vi "OuputMixer5782_500Mhz_2channel.vi"(6 "reset":bool, 8 "valid in":bool, 9 "Sine in":fxp<+/-,16,0>[](array[numeric])=[0.0, 0.0, 0.0, 0.0], 10 "Cosine in":fxp<+/-,16,0>[](array[numeric])=[0.0, 0.0, 0.0, 0.0], 11 "Data in":fxp<+/-,16,14>[](array[numeric])=[0.0, 0.0]) -> (0 "valid out":bool, 3 "appended array":i16[](array[numeric]))   [LabVIEW 2013]
doc: "Outputs input from channel 0 as I*cos(t)-Q*sin(t) on analog output 0"
uses:
  <vilib>/eio/EIONode/EIONode.xnode
  <vilib>/rvi/eio/common/nirviEmuTemplateMethod_errors.vi
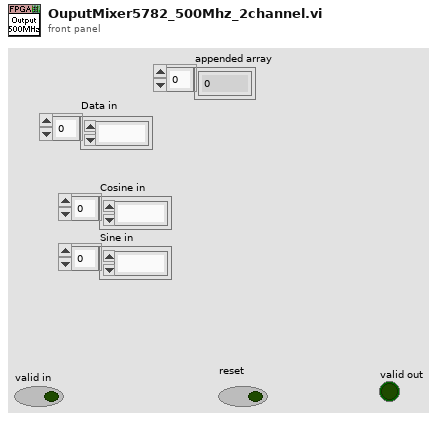
[diagram p1: front panel]
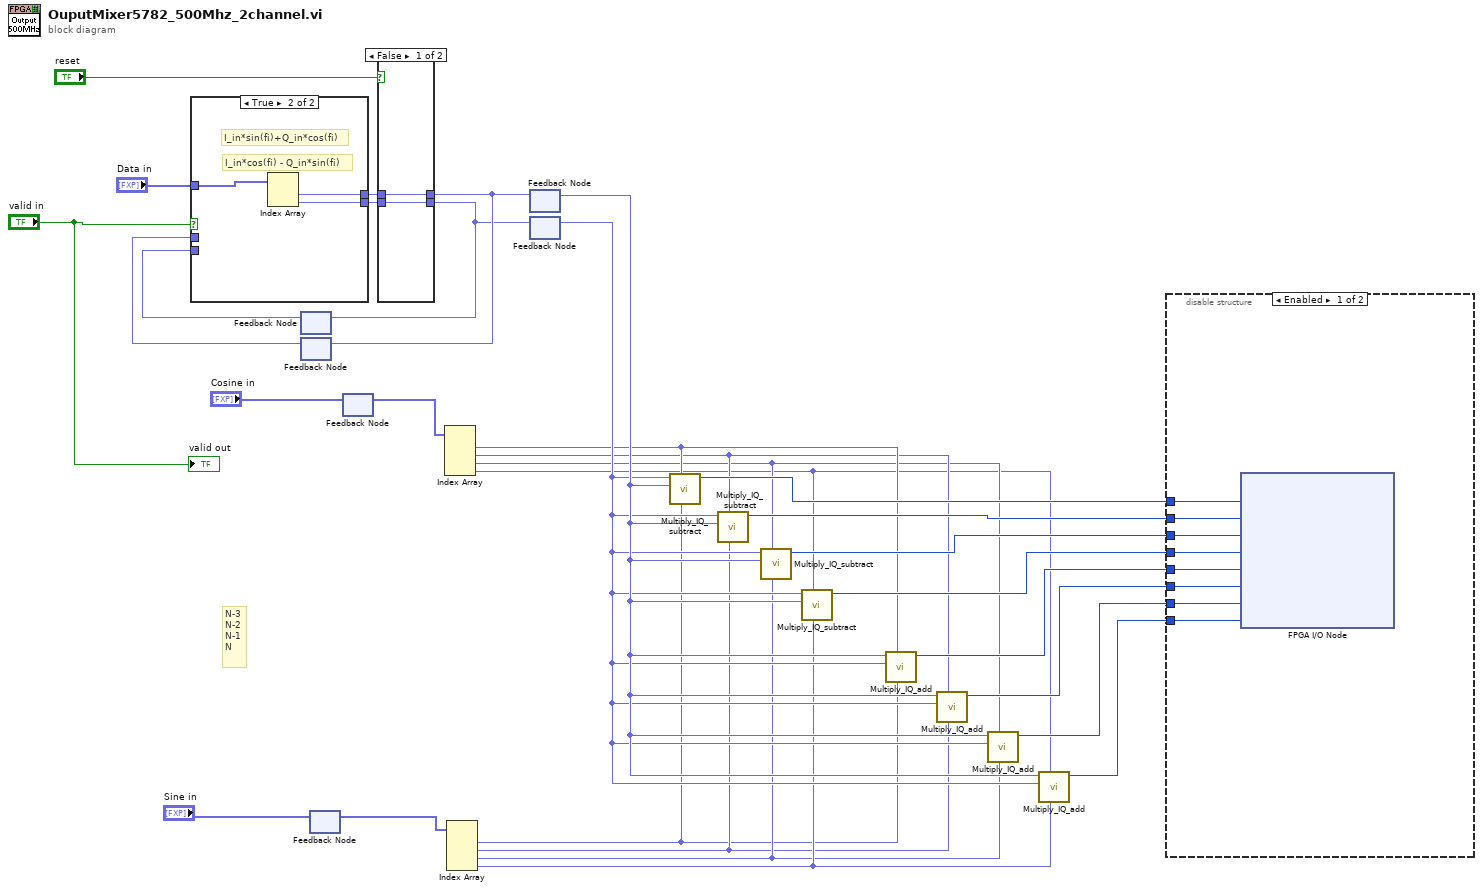
[diagram p0: block diagram]
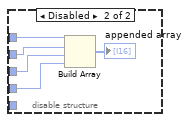
[diagram p2: hidden frame]
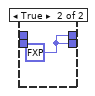
[diagram p3: hidden frame]
diagram:
  # "N-3\nN-2\nN-1\nN"
  n1 = feedback #1() -> (w29:fxp<+/-,16,14>)  [unwired: 1 in]
  n2 = feedback #2() -> (w28:fxp<+/-,16,14>)  [unwired: 1 in]
  n3 = case shown="True" "valid in" {
    tunnel: "Data in" -> [_ w36]
    tunnel: w29 -> [w32 _]
    tunnel: w28 -> [w33 _]
    tunnel: [w33 w35] -> w27
    tunnel: [w32 w34] -> w26
    frame False {
      # "keep old values"
    }
    frame True {
      # "I_in*cos(fi) - Q_in*sin(fi)"
      # "I_in*sin(fi)+Q_in*cos(fi)"
      n4 = Index Array(array=w36) -> (element #1=w35:fxp<+/-,16,14>, element #2=w34:fxp<+/-,16,14>)  [unwired: 2 in]
    }
  }
  n5 = feedback #3() -> (w25:fxp<+/-,16,0>[])  [unwired: 1 in]
  n6 = feedback-in #3("Sine in") -> ()
  n7 = feedback #4() -> (w24:fxp<+/-,16,0>[])  [unwired: 1 in]
  n8 = feedback-in #4("Cosine in") -> ()
  n9 = case shown="False" "reset" {
    tunnel: w27 -> [w37 _]
    tunnel: w26 -> [w38 _]
    tunnel: [w38 w39] -> w21
    tunnel: [w37 w39] -> w23
    frame False {
    }
    frame True {
      w39 = fxp<+/-,16,14> 0.0 ("Q in")
    }
  }
  n10 = feedback-in #1(w21) -> ()
  n11 = feedback-in #2(w23) -> ()
  n12 = Index Array(array=w24) -> (element #1=w9:fxp<+/-,16,0>, element #2=w8:fxp<+/-,16,0>, element #3=w7:fxp<+/-,16,0>, element #4=w6:fxp<+/-,16,0>)  [unwired: 4 in]
  n13 = Index Array(array=w25) -> (element #1=w2:fxp<+/-,16,0>, element #2=w3:fxp<+/-,16,0>, element #3=w4:fxp<+/-,16,0>, element #4=w5:fxp<+/-,16,0>)  [unwired: 4 in]
  n14 = feedback #5() -> (w22:fxp<+/-,16,14>)  [unwired: 1 in]
  n15 = feedback-in #5(w23) -> ()
  n16 = feedback #6() -> (w20:fxp<+/-,16,14>)  [unwired: 1 in]
  n17 = feedback-in #6(w21) -> ()
  n18 = call "Multiply_IQ_subtract.vi"("Sin"=w2, "Cos"=w9, "Q"=w22, "I"=w20) -> ("Z"=w17:i16)  [unwired: 6 in, 1 out]
  n19 = call "Multiply_IQ_subtract.vi"("Sin"=w3, "Cos"=w8, "Q"=w22, "I"=w20) -> ("Z"=w16:i16)  [unwired: 6 in, 1 out]
  n20 = call "Multiply_IQ_subtract.vi"("Sin"=w4, "Cos"=w7, "Q"=w22, "I"=w20) -> ("Z"=w15:i16)  [unwired: 6 in, 1 out]
  n21 = call "Multiply_IQ_subtract.vi"("Sin"=w5, "Cos"=w6, "Q"=w22, "I"=w20) -> ("Z"=w14:i16)  [unwired: 6 in, 1 out]
  n22 = call "Multiply_IQ_add.vi"("Sin"=w2, "Cos"=w9, "Q"=w20, "I"=w22) -> ("Z"=w13:i16)  [unwired: 6 in, 1 out]
  n23 = call "Multiply_IQ_add.vi"("Sin"=w3, "Cos"=w8, "Q"=w20, "I"=w22) -> ("Z"=w12:i16)  [unwired: 6 in, 1 out]
  n24 = call "Multiply_IQ_add.vi"("Sin"=w4, "Cos"=w7, "Q"=w20, "I"=w22) -> ("Z"=w11:i16)  [unwired: 6 in, 1 out]
  n25 = call "Multiply_IQ_add.vi"("Sin"=w5, "Cos"=w6, "Q"=w20, "I"=w22) -> ("Z"=w10:i16)  [unwired: 6 in, 1 out]
  n26 = disable-structure shown="Enabled" {
    disable-tunnel: w17 -> [w47 w52]
    disable-tunnel: w16 -> [w46 w51]
    disable-tunnel: w15 -> [w45 w50]
    disable-tunnel: w14 -> [w44 w49]
    disable-tunnel: w13 -> [w43 _]
    disable-tunnel: w12 -> [w42 _]
    disable-tunnel: w11 -> [w41 _]
    disable-tunnel: w10 -> [w40 _]
    frame Enabled {
      n27 = xnode "FPGA I/O Node"("IO Module\\AO 0 N-3"=w47, "IO Module\\AO 0 N-2"=w46, "IO Module\\AO 0 N-1"=w45, "IO Module\\AO 0 N"=w44, "IO Module\\AO 1 N-3"=w43, "IO Module\\AO 1 N-2"=w42, "IO Module\\AO 1 N-1"=w41, "IO Module\\AO 1 N"=w40) -> ()  [unwired: 8 in, 8 out]
    }
    frame Disabled {
      n28 = Build Array(w52, w51, w50, w49) -> (→"appended array":i16[])
    }
  }
  "valid out" <- "valid in"
